vi "Write to Info.vi"(6 "Additional Data":string, 7 "Write to Terminal":bool=TRUE, 8 "error in (no error)":errorcluster, 9 "gRPC Port":i32, 10 "Command":T1, 11 "Plugin Name":string) -> (0 "error out":errorcluster)   [LabVIEW 2021, in "CIFLogs.lvlib"]
uses:
  CIFLogs.lvlib
  Typedef/Plugin State Commands.ctl
  Typedef/Message Type.ctl
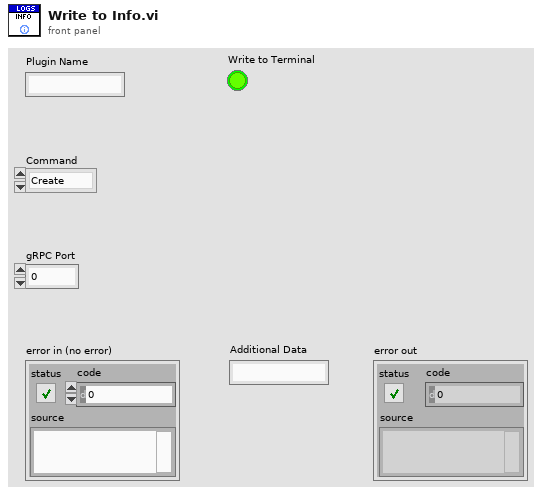
[diagram p1: front panel]
types:
  T1 = typedef "CIFLogs.lvlib/Plugin State Commands.ctl" = enum16{"Create", "Configure", "Run", "Pause", "Destroy", "Connect", "Force", "FIFO Instance"}
  T2 = typedef "CIFLogs.lvlib/Message Type.ctl" = enum16{"Error", "Information", "Print Terminal", "Configuration"}
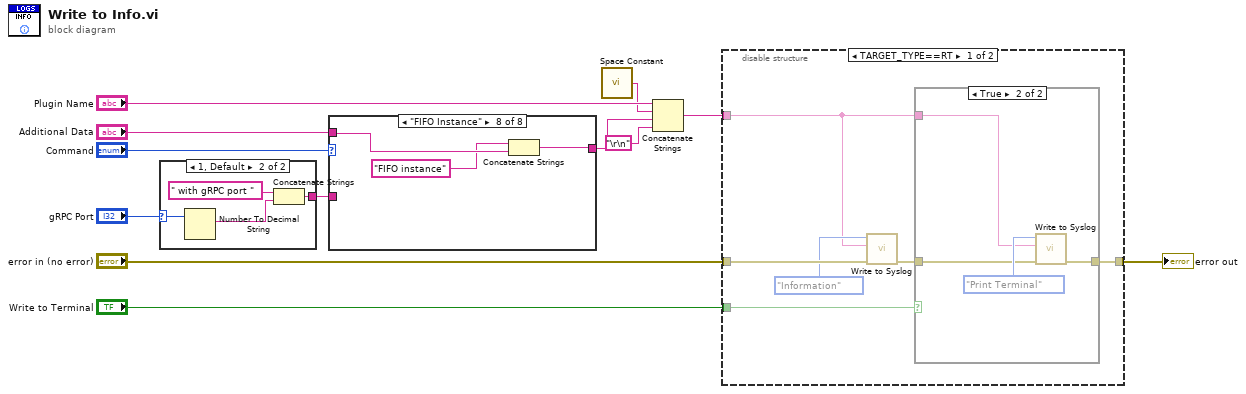
[diagram p0: block diagram]
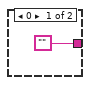
[diagram p2: hidden frame]
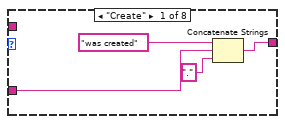
[diagram p3: hidden frame]
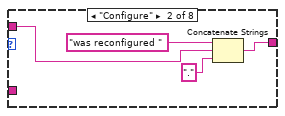
[diagram p4: hidden frame]
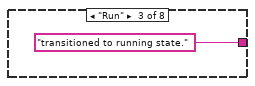
[diagram p5: hidden frame]
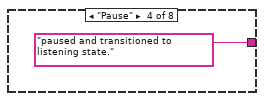
[diagram p6: hidden frame]
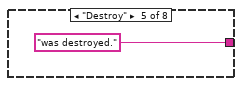
[diagram p7: hidden frame]
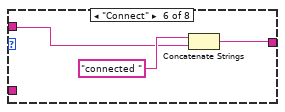
[diagram p8: hidden frame]
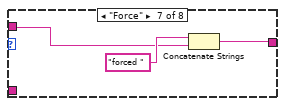
[diagram p9: hidden frame]
diagram:
  n1 = case shown="1, Default" "gRPC Port" {
    selector: "gRPC Port" -> [_ w17]
    tunnel: ["" w14] -> w3
    frame 0 {
    }
    frame 1, Default {
      n2 = Number To Decimal String(number=w17) -> (decimal integer string=w15:string)  [unwired: 1 in]
      n3 = Concatenate Strings(" with gRPC port ", w15) -> (w14:string)
    }
  }
  n4 = case shown="\"FIFO Instance\"" "Command" {
    tunnel: [w18 w23 "transitioned to running state." "paused and transitioned to listening state." "was destroyed." w29 w32 w36] -> w7
    tunnel: w3 -> [w20 _ _ _ _ _ _ _]
    tunnel: "Additional Data" -> [_ w22 _ _ _ w30 w33 w37]
    frame "Create" {
      n5 = Concatenate Strings("was created", w20, ".") -> (w18:string)
    }
    frame "Configure" {
      n6 = Concatenate Strings("was reconfigured ", w22, ".") -> (w23:string)
    }
    frame "Run" {
    }
    frame "Pause" {
    }
    frame "Destroy" {
    }
    frame "Connect" {
      n7 = Concatenate Strings("connected ", w30) -> (w29:string)
    }
    frame "Force" {
      n8 = Concatenate Strings("forced ", w33) -> (w32:string)
    }
    frame "FIFO Instance" {
      n9 = Concatenate Strings("FIFO instance", w37) -> (w36:string)
    }
  }
  n10 = call <vilib>:"Space Constant.vi"() -> ("String"=w6:string)
  n11 = Concatenate Strings("Plugin Name", w6, w7, "\r\n") -> (w9:string)
  n12 = disable-structure shown="TARGET_TYPE==RT" {
    disable-tunnel: "error in (no error)" -> [w42 _]
    disable-tunnel: [w43 _] -> w11
    disable-tunnel: w9 -> [w39 _]
    disable-tunnel: "Write to Terminal" -> [w38 _]
    frame condition #0 {
      n13 = call "Write to Syslog.vi"("error in (no error)"=w42, "message"=w39, "CIF Message Type"=Message_Type."Information") -> ("error out"=w41:errorcluster)  [unwired: 8 in]
      n14 = case shown="True" w38 {
        tunnel: [w44 w48] -> w43
        tunnel: w41 -> [w44 w46]
        tunnel: w39 -> [_ w45]
        frame False {
        }
        frame True {
          n15 = call "Write to Syslog.vi"("error in (no error)"=w46, "message"=w45, "CIF Message Type"=Message_Type."Print Terminal") -> ("error out"=w48:errorcluster)  [unwired: 8 in]
        }
      }
    }
    frame condition #1 (active) {
    }
  }
  "error out" <- w11
